vi "Set Attacked.vi"(9 "Column":i32, 10 "Row":i32, 11 "Temp DVR":refnum<data-value>) -> (3 "Temp DVR":refnum<data-value>)   [LabVIEW 2014, in "SquareBattle.lvclass"]
uses:
  SquareBattle.lvclass
  Runner Cluster.ctl
  Runner/Runner.lvclass
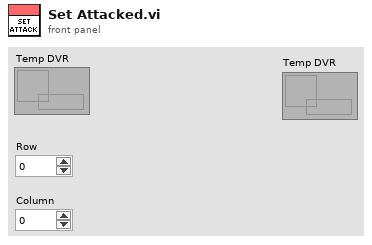
[diagram p1: front panel]
types:
  T1 = typedef "SquareBattle.lvclass/Runner Cluster.ctl" = cluster{"Attacked?":bool, "DVR":refnum<data-value>, "Team":i32, "Player":i32, "Next Turn":i32}
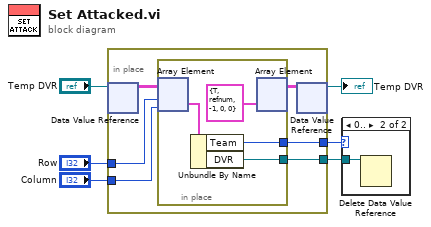
[diagram p0: block diagram]
diagram:
  n1 = in-place {
    in-place-border: "Row" -> [w11]
    in-place-border: "Column" -> [w10]
    in-place-border: [w8] -> w2
    in-place-border: [w7] -> w1
    n2 = in-place-dvr #1("Temp DVR") -> (w12:T1[][])  [unwired: 1 out]
    n3 = in-place {
      in-place-border: [w14] -> w8
      in-place-border: [w13] -> w7
      n4 = in-place-array #2(w12, w11, w10) -> (w16:T1)
      n5 = Unbundle By Name(w16) -> ("Team"=w14:i32, "DVR"=w13:refnum<data-value>)
      n6 = in-place-array #2(T1 {"Attacked?"=TRUE, "DVR"=refnum, "Team"=-1, "Player"=0, "Next Turn"=0} ("Cluster")) -> (w9:T1[][])  [unwired: 2 out]
    }
    n7 = in-place-dvr #1(w9) -> (→"Temp DVR":refnum<data-value>)  [unwired: 1 out]
  }
  n8 = case shown="0.." w2 {
    tunnel: w1 -> [_ w17]
    frame ..-1 {
    }
    frame 0.. {
      n9 = Delete Data Value Reference(data value reference=w17) -> ()  [unwired: 1 in, 2 out]
    }
  }
